vi "Render Point Defense.vi"(7 "Renderer":refnum<class "Renderer.lvclass">, 8 "error in (no error)":errorcluster, 10 "Camera":refnum<class "Camera.lvclass">, 11 "Chmmr in":refnum<class "Chmmr.lvclass">) -> (0 "error out":errorcluster)   [LabVIEW 2026]
uses:
  Chmmr.lvclass
  C:/dev/LabVIEW/LabMelee/Source/Application Specific/Element/Element.lvclass
  Camera/Camera.lvclass
  Renderer/Renderer.lvclass
  Element/Element.lvclass/Element.ctl
  Motion/Motion.lvclass/Motion.ctl
  Chmmr.lvclass/Chmmr.ctl
  Deployables/Zap Sat/Zap Sat.lvclass/Zap Sat.ctl
  C:/dev/LabVIEW/LabMelee/Source/Application Specific/Ship/Ship.lvclass
  C:/dev/LabVIEW/LabMelee/Source/Application Specific/Ships/Chmmr/Chmmr.lvclass
  Vector 2D/Vector 2D.lvclass
  Deployables/Zap Sat/Zap Sat.lvclass
  C:/dev/LabVIEW/LabMelee/Source/Application Specific/Deployable/Deployable.lvclass
  C:/dev/LabVIEW/LabMelee/Source/Application Specific/Deployables/Zap Sat/Zap Sat.lvclass
  LabSDL2/Source/Libraries/LibSDL2 Wrapper/LibSDL2.lvlib
  Element/Element.lvclass
  LabSDL2/Source/Libraries/SDL2 Utility/Point (I32).ctl
  LabSDL2/Source/Libraries/SDL2 Utility/SDL2 Utility.lvlib
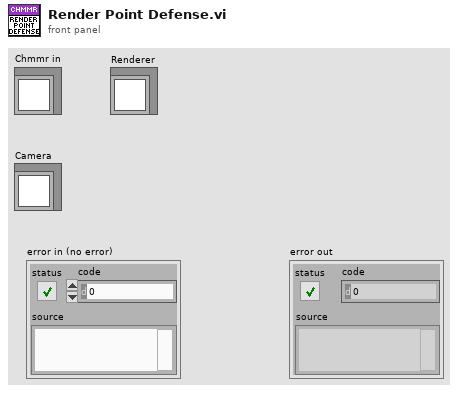
[diagram p1: front panel]
types:
  T1 = typedef "SDL2 Utility.lvlib/Point (I32).ctl" = cluster{"x":i32, "y":i32}
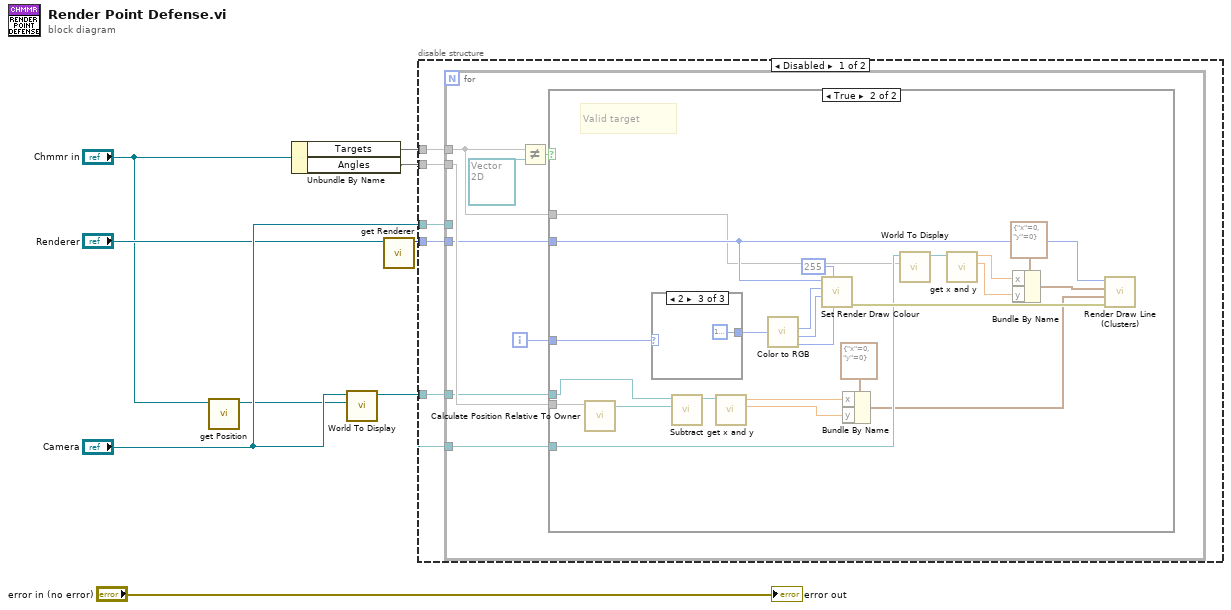
[diagram p0: block diagram]
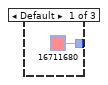
[diagram p3: hidden frame]
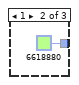
[diagram p4: hidden frame]
diagram:
  n1 = call "get Position.vi"("Element in"="Chmmr in") -> ("Position"=w1:refnum<class "Vector 2D.lvclass">)  [unwired: 10 in]
  n2 = Unbundle By Name("Chmmr in") -> ("Targets"=w9, "Angles"=w8)
  n3 = call "World To Display.vi"("World Position"=w1, "Camera in"="Camera") -> ("Display Position"=w6:refnum<class "Vector 2D.lvclass">)  [unwired: 9 in]
  n4 = call-dynamic "get Renderer.vi"("Renderer in"="Renderer") -> ("Renderer"=w3:u32)  [unwired: 10 in]
  n5 = disable-structure shown="Disabled" {
    disable-tunnel: w9 -> [w14 _]
    disable-tunnel: w8 -> [w13 _]
    disable-tunnel: "Camera" -> [w12 _]
    disable-tunnel: w6 -> [w11 _]
    disable-tunnel: w3 -> [w10 _]
    frame Disabled {
      n6 = for {
        tunnel: w14 -> [w22]
        tunnel: w12 -> [_]
        tunnel: w10 -> [w19]
        tunnel: w13 -> [w21]
        tunnel: w12 -> [w17]
        tunnel: w11 -> [w20]
        i -> [w18]
        n7 = Not Equal?(x=w22, y=refnum<class "Vector 2D.lvclass"> refnum ("Vector 2D out")) -> (x != y?=w16:bool)
        n8 = case shown="True" w16 {
          tunnel: w22 -> [_ w33]
          tunnel: w21 -> [_ w45]
          tunnel: w20 -> [_ w35]
          tunnel: w19 -> [_ w42]
          tunnel: w18 -> [_ w41]
          tunnel: w17 -> [_ w40]
          frame False {
            # "No target"
          }
          frame True {
            # "Valid target"
            n9 = call "Calculate Position Relative To Owner.vi"("Zap Sat in"=w45) -> ("Position"=w34:refnum<class "Vector 2D.lvclass">)  [unwired: 10 in]
            n10 = case shown="2" w41 {
              tunnel: [u32 16711680 ("Color") u32 6618880 u32 16777224] -> w36
              frame Default {
              }
              frame 1 {
              }
              frame 2 {
              }
            }
            n11 = call "Subtract.vi"("B"=w34, "A"=w35) -> ("A-B"=w25:refnum<class "Vector 2D.lvclass">)  [unwired: 9 in]
            n12 = call "get x and y.vi"("Vector 2D in"=w25) -> ("y"=w24:sgl, "x"=w27:sgl)  [unwired: 9 in]
            n13 = call <vilib>:"Color to RGB.vi"("Color"=w36) -> ("R"=w39:u8, "G"=w38:u8, "B"=w37:u8)  [unwired: 1 out]
            n14 = call "Set Render Draw Colour.vi"("B"=w37, "A"=u8 255, "G"=w38, "R"=w39, "Renderer Pointer"=w42) -> ("error out"=w43:errorcluster)  [unwired: 5 in, 1 out]
            n15 = Bundle By Name(cluster=T1 {"x"=0, "y"=0} ("Start"), "x"=w27, "y"=w24) -> (w23:T1)
            n16 = call "World To Display.vi"("World Position"=w33, "Camera in"=w40) -> ("Display Position"=w32:refnum<class "Vector 2D.lvclass">)  [unwired: 9 in]
            n17 = call "get x and y.vi"("Vector 2D in"=w32) -> ("y"=w28:sgl, "x"=w29:sgl)  [unwired: 9 in]
            n18 = Bundle By Name(cluster=T1 {"x"=0, "y"=0} ("Start"), "x"=w29, "y"=w28) -> (w30:T1)
            n19 = call "Render Draw Line (Clusters).vi"("error in"=w43, "End"=w23, "Start"=w30, "Renderer Pointer"=w42) -> ()  [unwired: 6 in, 2 out]
          }
        }
      }
    }
    frame Enabled {
    }
  }
  "error out" <- "error in (no error)"
